vi "Set Output Actor NRQ.vi"(8 "error in (no error)":errorcluster, 10 "Actor Framework:Message Enqueuer":refnum<class "Message Enqueuer.lvclass">, 11 "output_poller_actor in":refnum<class "output_poller_actor.lvclass">) -> (0 "error out":errorcluster, 3 "output_poller_actor out":refnum<class "output_poller_actor.lvclass">)   [LabVIEW 2015, in "output_poller_actor.lvclass"]
uses:
  output_poller_actor.lvclass
  <vilib>/ActorFramework/Message Enqueuer/Message Enqueuer.lvclass
  output_poller_actor.lvclass/output_poller_actor.ctl
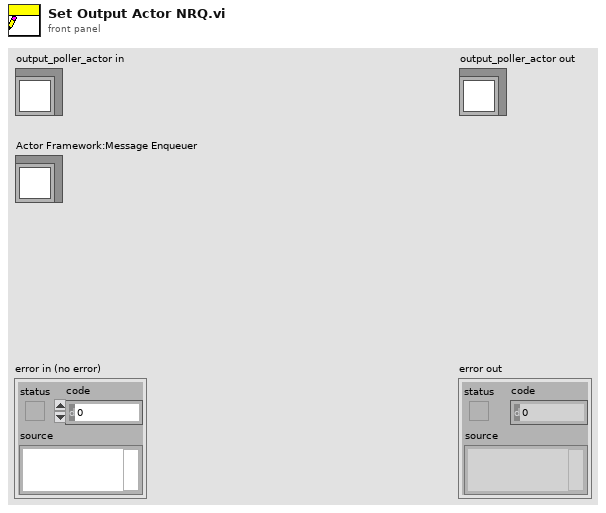
[diagram p1: front panel]
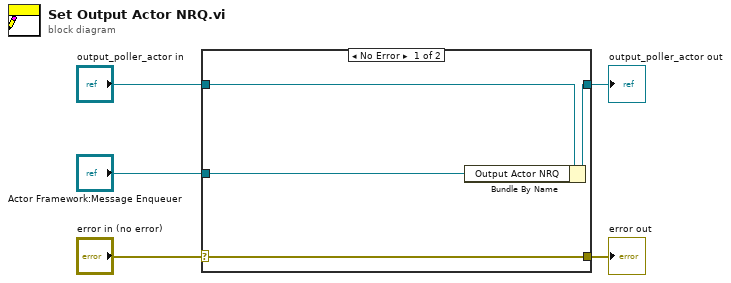
[diagram p0: block diagram]
diagram:
  n1 = case shown="No Error" "error in (no error)" {
    selector: "error in (no error)" -> [w9 w10]
    tunnel: [w9 w10] -> w4
    tunnel: [w7 w11] -> w2
    tunnel: "output_poller_actor in" -> [w8 w11]
    tunnel: "Actor Framework:Message Enqueuer" -> [w6 _]
    frame No Error {
      n2 = Bundle By Name(cluster=w8, "Output Actor NRQ"=w6) -> (w7:refnum<class "output_poller_actor.lvclass">)
    }
    frame Error {
    }
  }
  "error out" <- w4
  "output_poller_actor out" <- w2
